vi "yolov8_postprocess.vi"(5 "nms_threshold":sgl=0.4, 6 "use letterbox":bool=TRUE, 7 "confThreshold":sgl=0.5, 8 "error in (no error)":errorcluster, 10 "2d_data":sgl[][](array[numeric]), 11 "image":refnum<class "Mat_8U.lvclass">) -> (0 "error out":errorcluster, 2 "results":T2, 3 "reference out":refnum<class "Mat_8U.lvclass">)   [LabVIEW 2023]
uses:
  <vilib>/addons/VIRobotics/opencv_yiku/Mat/Mat_8U/Mat_8U.lvclass
  C:/Program Files/National Instruments/LabVIEW 2023/vi.lib/addons/VIRobotics/opencv_yiku/Mat/Mat/Mat.lvclass
  <vilib>/addons/VIRobotics/opencv_yiku/ctls/Rect.ctl
  <vilib>/addons/VIRobotics/opencv_yiku/opencv_yiku.lvlib
panel:
  out "Array":T1[](array[typedef])
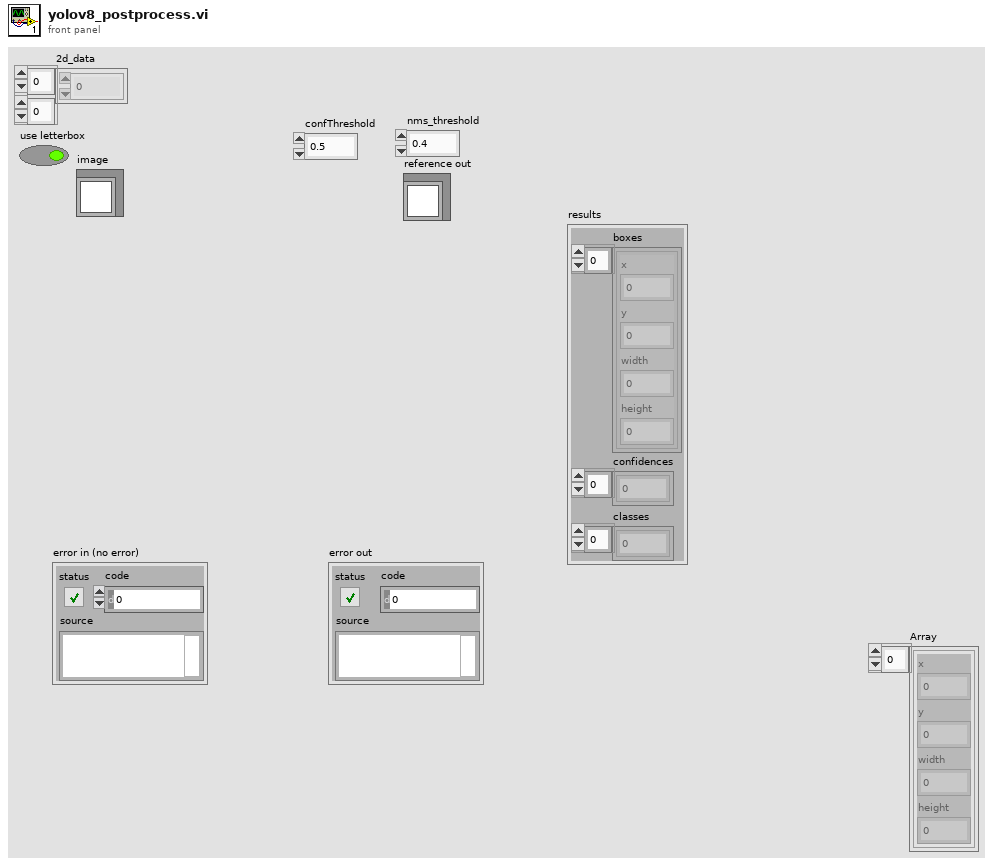
[diagram p1: front panel]
types:
  T1 = typedef "opencv_yiku.lvlib/Rect.ctl" = cluster{"x":i32, "y":i32, "width":i32, "height":i32}
  T2 = cluster{"boxes":T1[], "confidences":sgl[], "classes":i32[]}
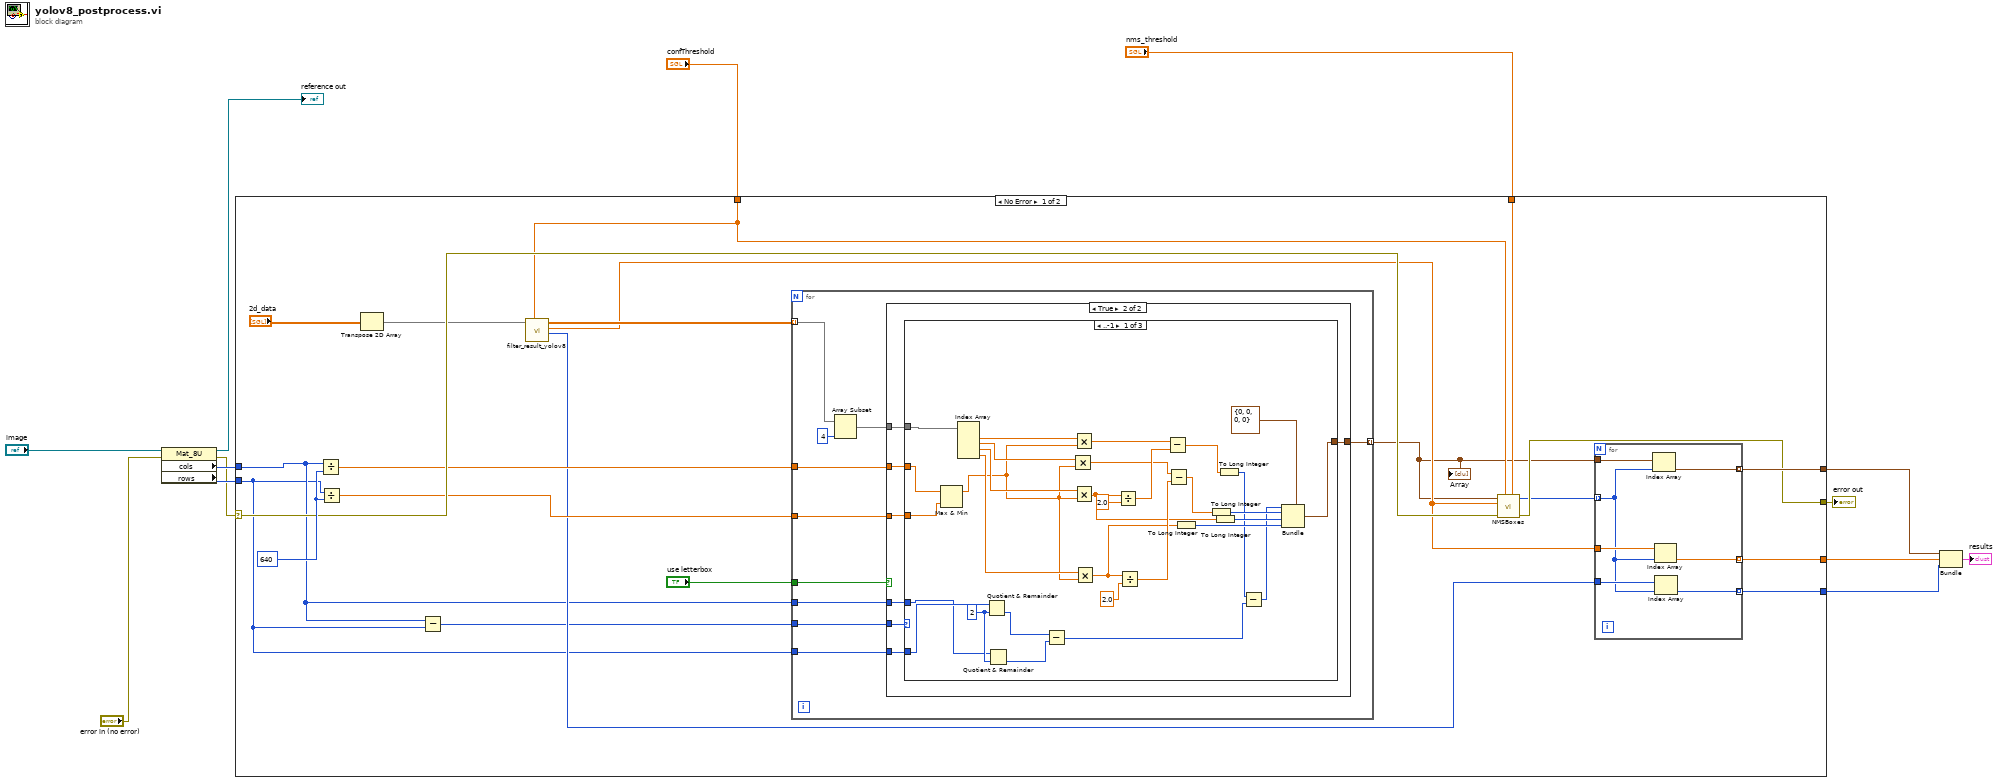
[diagram p0: block diagram]
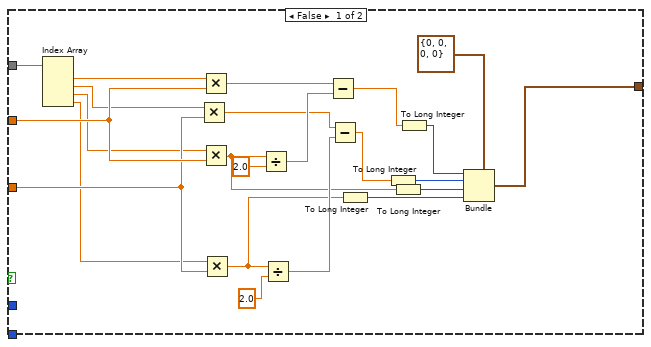
[diagram p2: hidden frame]
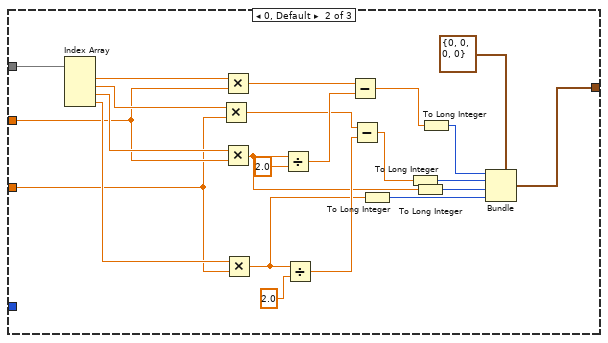
[diagram p3: hidden frame]
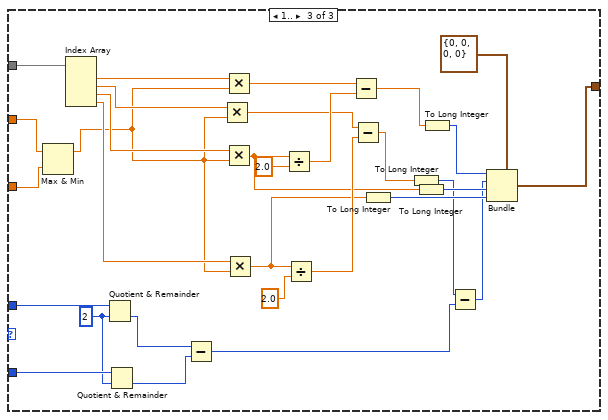
[diagram p4: hidden frame]
diagram:
  n1 = property class="Mat_8U"(reference="image", error in="error in (no error)") -> (reference out=→"reference out":refnum<class "Mat_8U.lvclass">, error out=w7:errorcluster, "cols"=w10:i32, "rows"=w11:i32)
  n2 = case shown="No Error" w7 {
    selector: w7 -> [w28 w167]
    tunnel: [w34 _] -> w3
    tunnel: [w33 _] -> w4
    tunnel: [w32 _] -> w5
    tunnel: "nms_threshold" -> [w31 _]
    tunnel: "confThreshold" -> [w23 _]
    tunnel: w11 -> [w16 _]
    tunnel: w10 -> [w17 _]
    tunnel: [w30 w167] -> w6
    frame No Error {
      w29 = 640 ("y")
      n3 = Divide(x=w17, y=w29) -> (x/y=w26:dbl)
      n4 = Divide(x=w16, y=w29) -> (x/y=w25:dbl)
      n5 = Transpose 2D Array(2D array="2d_data") -> (transposed array=w14:sgl[][])
      n6 = Subtract(x=w17, y=w16) -> (x-y=w18:i32)
      n7 = call "filter_result_yolov8.vi"("confThreshold"=w23, "2d_data"=w14) -> ("index"=w21:i32[], "scores"=w22:sgl[], "filtered_data"=w24:sgl[][])  [unwired: 7 in]
      n8 = for {
        tunnel: w24 -> [w42] mode=indexing
        tunnel: w26 -> [w44]
        tunnel: w25 -> [w43]
        tunnel: [w39] -> w20 mode=indexing
        tunnel: "use letterbox" -> [w38]
        tunnel: w18 -> [w37]
        tunnel: w17 -> [w36]
        tunnel: w16 -> [w35]
        n9 = Array Subset(array=w42, length=4) -> (w40:sgl[])  [unwired: 1 in]
        n10 = case shown="True" w38 {
          tunnel: w44 -> [w67 w73]
          tunnel: w43 -> [w66 w72]
          tunnel: w40 -> [w65 w71]
          tunnel: [w45 w70] -> w39
          tunnel: w37 -> [_ w74]
          tunnel: w36 -> [_ w69]
          tunnel: w35 -> [_ w68]
          frame False {
            n11 = Index Array(array=w65) -> (element #1=w64:sgl, element #2=w63:sgl, element #3=w62:sgl, element #4=w61:sgl)  [unwired: 4 in]
            n12 = Multiply(x=w63, y=w66) -> (x*y=w56:dbl)
            n13 = Multiply(x=w64, y=w67) -> (x*y=w58:dbl)
            n14 = Multiply(x=w62, y=w67) -> (x*y=w51:dbl)
            n15 = Multiply(x=w61, y=w66) -> (x*y=w53:dbl)
            n16 = Divide(x=w51, y=sgl 2.0) -> (x/y=w57:dbl)
            n17 = Divide(x=w53, y=sgl 2.0) -> (x/y=w55:dbl)
            n18 = Subtract(x=w58, y=w57) -> (x-y=w47:dbl)
            n19 = Subtract(x=w56, y=w55) -> (x-y=w49:dbl)
            n20 = To Long Integer(number=w53) -> (32bit integer=w52:i32)
            n21 = To Long Integer(number=w49) -> (32bit integer=w48:i32)
            n22 = To Long Integer(number=w51) -> (32bit integer=w50:i32)
            n23 = To Long Integer(number=w47) -> (32bit integer=w46:i32)
            n24 = Bundle(cluster=T1 {"x"=0, "y"=0, "width"=0, "height"=0} ("Rect"), "x"=w46, "y"=w48, "width"=w50, "height"=w52) -> (w45:T1)
          }
          frame True {
            n25 = case shown="..-1" w74 {
              tunnel: w73 -> [w76 w109 w132]
              tunnel: w72 -> [w75 w108 w131]
              tunnel: w71 -> [w83 w107 w141]
              tunnel: [w82 w106 w140] -> w70
              tunnel: w69 -> [w80 _ w139]
              tunnel: w68 -> [w81 _ w138]
              frame ..-1 {
                w88 = 2 ("y")
                n26 = Max & Min(x=w76, y=w75) -> (max(x,y)=w84:dbl)  [unwired: 1 out]
                n27 = Index Array(array=w83) -> (element #1=w105:sgl, element #2=w104:sgl, element #3=w103:sgl, element #4=w102:sgl)  [unwired: 4 in]
                n28 = Quotient & Remainder(x=w81, y=w88) -> (floor(x/y)=w87:i32)  [unwired: 1 out]
                n29 = Quotient & Remainder(x=w80, y=w88) -> (floor(x/y)=w86:i32)  [unwired: 1 out]
                n30 = Subtract(x=w87, y=w86) -> (x-y=w85:i32)
                n31 = Multiply(x=w104, y=w84) -> (x*y=w97:dbl)
                n32 = Multiply(x=w105, y=w84) -> (x*y=w99:dbl)
                n33 = Multiply(x=w103, y=w84) -> (x*y=w92:dbl)
                n34 = Multiply(x=w102, y=w84) -> (x*y=w94:dbl)
                n35 = Divide(x=w92, y=sgl 2.0) -> (x/y=w98:dbl)
                n36 = Divide(x=w94, y=sgl 2.0) -> (x/y=w96:dbl)
                n37 = Subtract(x=w99, y=w98) -> (x-y=w89:dbl)
                n38 = Subtract(x=w97, y=w96) -> (x-y=w90:dbl)
                n39 = To Long Integer(number=w94) -> (32bit integer=w93:i32)
                n40 = To Long Integer(number=w90) -> (32bit integer=w79:i32)
                n41 = To Long Integer(number=w92) -> (32bit integer=w91:i32)
                n42 = To Long Integer(number=w89) -> (32bit integer=w78:i32)
                n43 = Subtract(x=w78, y=w85) -> (x-y=w77:i32)
                n44 = Bundle(cluster=T1 {"x"=0, "y"=0, "width"=0, "height"=0} ("Rect"), "x"=w77, "y"=w79, "width"=w91, "height"=w93) -> (w82:T1)
              }
              frame 0, Default {
                n45 = Index Array(array=w107) -> (element #1=w128:sgl, element #2=w127:sgl, element #3=w126:sgl, element #4=w125:sgl)  [unwired: 4 in]
                n46 = Multiply(x=w127, y=w108) -> (x*y=w120:dbl)
                n47 = Multiply(x=w128, y=w109) -> (x*y=w122:dbl)
                n48 = Multiply(x=w126, y=w109) -> (x*y=w115:dbl)
                n49 = Multiply(x=w125, y=w108) -> (x*y=w117:dbl)
                n50 = Divide(x=w115, y=sgl 2.0) -> (x/y=w121:dbl)
                n51 = Divide(x=w117, y=sgl 2.0) -> (x/y=w119:dbl)
                n52 = Subtract(x=w122, y=w121) -> (x-y=w111:dbl)
                n53 = Subtract(x=w120, y=w119) -> (x-y=w113:dbl)
                n54 = To Long Integer(number=w117) -> (32bit integer=w116:i32)
                n55 = To Long Integer(number=w113) -> (32bit integer=w112:i32)
                n56 = To Long Integer(number=w115) -> (32bit integer=w114:i32)
                n57 = To Long Integer(number=w111) -> (32bit integer=w110:i32)
                n58 = Bundle(cluster=T1 {"x"=0, "y"=0, "width"=0, "height"=0} ("Rect"), "x"=w110, "y"=w112, "width"=w114, "height"=w116) -> (w106:T1)
              }
              frame 1.. {
                w137 = 2 ("y")
                n59 = Max & Min(x=w132, y=w131) -> (max(x,y)=w130:dbl)  [unwired: 1 out]
                n60 = Index Array(array=w141) -> (element #1=w159:sgl, element #2=w158:sgl, element #3=w157:sgl, element #4=w156:sgl)  [unwired: 4 in]
                n61 = Quotient & Remainder(x=w139, y=w137) -> (floor(x/y)=w136:i32)  [unwired: 1 out]
                n62 = Quotient & Remainder(x=w138, y=w137) -> (floor(x/y)=w135:i32)  [unwired: 1 out]
                n63 = Subtract(x=w136, y=w135) -> (x-y=w134:i32)
                n64 = Multiply(x=w158, y=w130) -> (x*y=w151:dbl)
                n65 = Multiply(x=w159, y=w130) -> (x*y=w153:dbl)
                n66 = Multiply(x=w157, y=w130) -> (x*y=w146:dbl)
                n67 = Multiply(x=w156, y=w130) -> (x*y=w148:dbl)
                n68 = Divide(x=w146, y=sgl 2.0) -> (x/y=w152:dbl)
                n69 = Divide(x=w148, y=sgl 2.0) -> (x/y=w150:dbl)
                n70 = Subtract(x=w153, y=w152) -> (x-y=w143:dbl)
                n71 = Subtract(x=w151, y=w150) -> (x-y=w144:dbl)
                n72 = To Long Integer(number=w148) -> (32bit integer=w147:i32)
                n73 = To Long Integer(number=w144) -> (32bit integer=w133:i32)
                n74 = To Long Integer(number=w146) -> (32bit integer=w145:i32)
                n75 = To Long Integer(number=w143) -> (32bit integer=w142:i32)
                n76 = Subtract(x=w133, y=w134) -> (x-y=w129:i32)
                n77 = Bundle(cluster=T1 {"x"=0, "y"=0, "width"=0, "height"=0} ("Rect"), "x"=w142, "y"=w129, "width"=w145, "height"=w147) -> (w140:T1)
              }
            }
          }
        }
      }
      "Array" <- w20
      n78 = call <vilib>:"NMSBoxes.vi"("nms_threshold"=w31, "score_threshold"=w23, "error in (no error)"=w28, "scores"=w22, "boxes"=w20) -> ("error out"=w30:errorcluster, "result"=w27:i32[])  [unwired: 5 in]
      n79 = for {
        tunnel: w27 -> [w163] mode=indexing
        tunnel: w20 -> [w166]
        tunnel: w22 -> [w165]
        tunnel: w21 -> [w164]
        tunnel: [w162] -> w32 mode=indexing
        tunnel: [w161] -> w33 mode=indexing
        tunnel: [w160] -> w34 mode=indexing
        n80 = Index Array(array=w166, index=w163) -> (element=w162:T1)
        n81 = Index Array(array=w165, index=w163) -> (element=w161:sgl)
        n82 = Index Array(array=w164, index=w163) -> (element=w160:i32)
      }
    }
    frame Error {
    }
  }
  "error out" <- w6
  n83 = Bundle(w5, w4, w3) -> (→"results":cluster{T1[], sgl[], i32[]})  [unwired: 1 in]
